vi "rx streamer max num samps.vi"(8 "error in (no error)":errorcluster, 10 "max_num_samps_out":u64, 11 "h":u64) -> (0 "error out":errorcluster, 1 "max_num_samps_out out":u64, 2 "function return":u32(ring), 3 "h 2":u64)   [LabVIEW 2023, in "uhd.lvlib"]
doc: "UHD_API uhd_error uhd_rx_streamer_max_num_samps(\n uhd_rx_streamer_handle h, size_t* max_num_samps_out);"
uses:
  <userlib>/uhd/uhd.lvlib
  <userlib>/uhd/uhd.dll
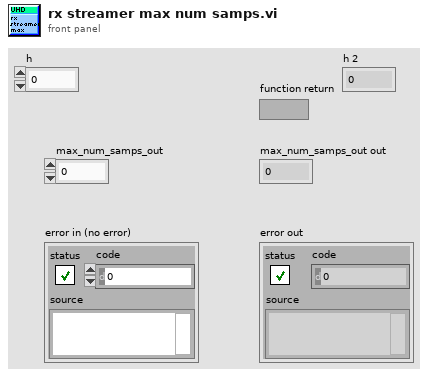
[diagram p1: front panel]
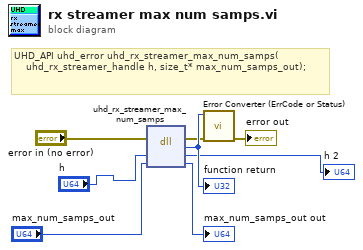
[diagram p0: block diagram]
diagram:
  # "UHD_API uhd_error uhd_rx_streamer_max_num_samps(\n    uhd_rx_streamer_handle h, size_t* max_num_samps_out);"
  n1 = dll-call lib="C:/Program Files/National Instruments/LabVIEW 2023/user.lib/uhd/uhd.dll" fn="uhd_rx_streamer_max_num_samps"(error in="error in (no error)", "h"="h", "max_num_samps_out"="max_num_samps_out") -> (error out=w4:errorcluster, "return type"=w8:u32, "h"=→"h 2":u64, "max_num_samps_out"=→"max_num_samps_out out":u64)  [unwired: 2 in, 1 out]
  "function return" <- w8
  n2 = call <userlib>:"Error Converter (ErrCode or Status).vi"("error in (no error)"=w4, "error code"=w8) -> ("error out"=→"error out":errorcluster)  [unwired: 9 in]
